vi "Get Routine Object.vi"(7 "Settings":T2=enum."Custom", 8 "error in (no error)":errorcluster, 11 "Routine":T1=enum."Secure Syringe") -> (0 "error out":errorcluster, 3 "Routine out":refnum<class "Routine.lvclass">)   [LabVIEW 2020, in "Routine.lvclass"]
uses:
  Routine.lvclass
  Pick and Place/Pick and Place.lvclass
  Pick and Place/Pick and Place Type.ctl
  Secure Syringe/SecureRelease Syringe.lvclass
  Settings.ctl
  Projects/Sensor Dispense.lvclass
  Dispense/Iterative Dispense/Iterative Dispense.lvclass
  Routine Enum.ctl
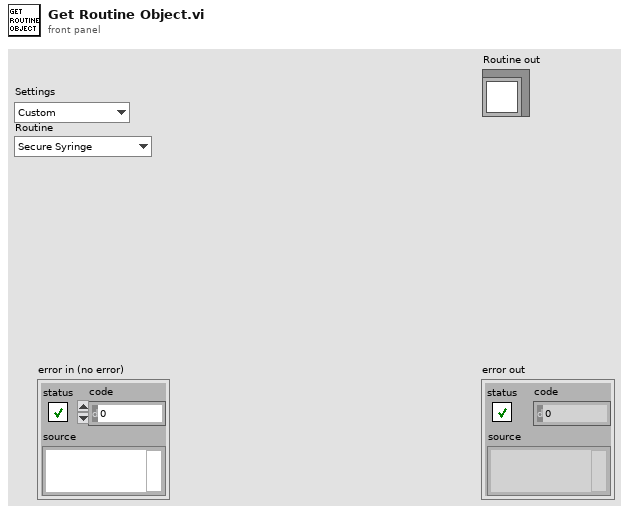
[diagram p1: front panel]
types:
  T1 = typedef "Routine.lvclass/Routine Enum.ctl" = enum16{"Primary Pick Up", "Pick Up All", "Put Down Secondary", "Put Down All", "Release Syringe", "Secondary Pick Up", "Secure Syringe", "Dispense on Plate", "Dispense on Kapton", "Dispense on Sensor"}
  T2 = typedef "Routine.lvclass/Settings.ctl" = enum16{"Default", "Custom"}
  T3 = typedef "Pick and Place.lvclass/Pick and Place Type.ctl" = enum16{"Primary Pick Up", "Secondary Pick Up", "Put Down All", "Pick Up All", "Put Down Secondary"}
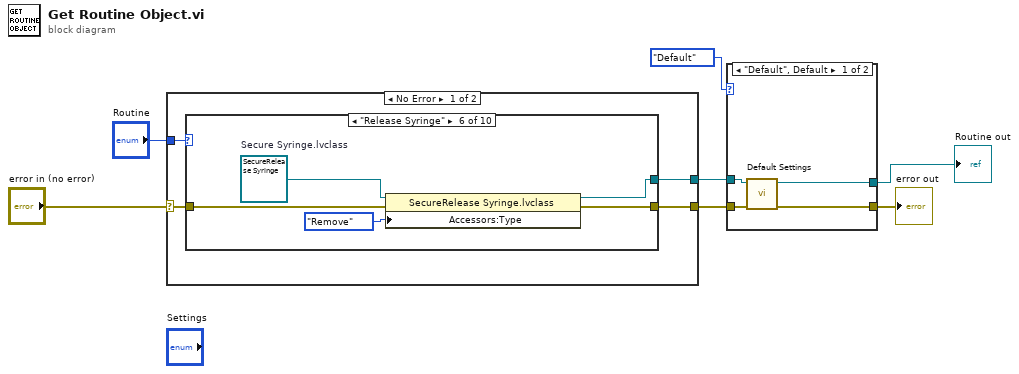
[diagram p0: block diagram]
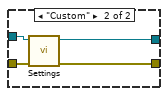
[diagram p2: hidden frame]
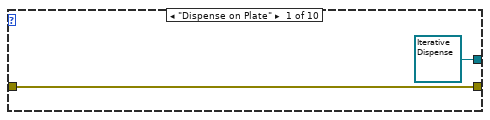
[diagram p3: hidden frame]
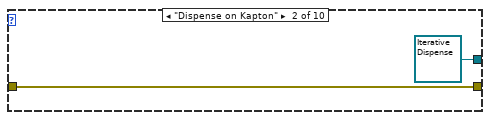
[diagram p4: hidden frame]
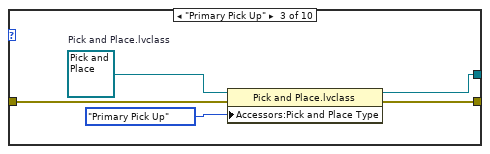
[diagram p5: hidden frame]
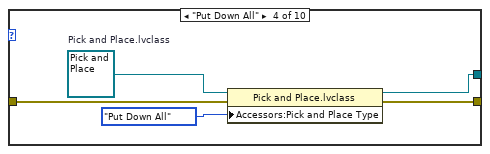
[diagram p6: hidden frame]
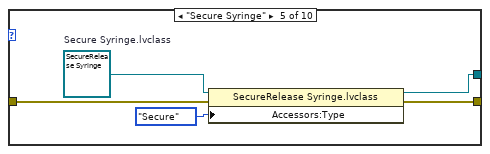
[diagram p7: hidden frame]
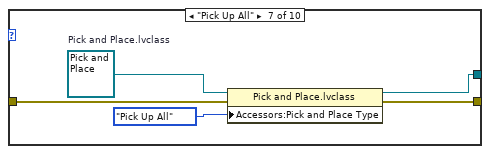
[diagram p8: hidden frame]
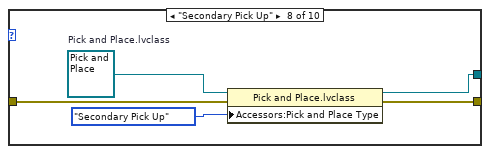
[diagram p9: hidden frame]
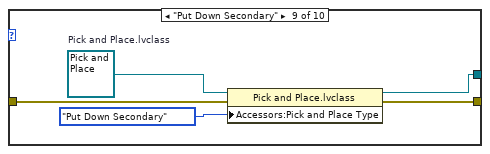
[diagram p10: hidden frame]
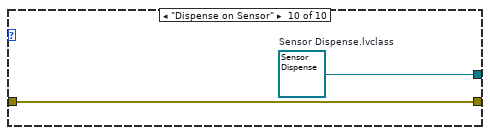
[diagram p11: hidden frame]
diagram:
  n1 = case shown="No Error" "error in (no error)" {
    selector: "error in (no error)" -> [w9 w53]
    tunnel: [w8 w53] -> w2
    tunnel: [w11 _] -> w6
    tunnel: "Routine" -> [w10 _]
    frame No Error {
      n2 = case shown="\"Release Syringe\"" w10 {
        tunnel: [refnum<class "Iterative Dispense.lvclass"> refnum ("Iterative Dispense.lvclass") refnum<class "Iterative Dispense.lvclass"> refnum ("Iterative Dispense.lvclass") w19 w24 w28 w33 w38 w43 w48 w52] -> w11
        tunnel: w9 -> [w13 w15 w17 w22 w27 w32 w37 w42 w47 w51]
        tunnel: [w13 w15 w16 w21 w26 w31 w36 w41 w46 w51] -> w8
        frame "Dispense on Plate" {
        }
        frame "Dispense on Kapton" {
        }
        frame "Primary Pick Up" {
          w20 = refnum<class "Pick and Place.lvclass"> refnum  # Pick and Place.lvclass
          n3 = property class="Pick and Place.lvclass"(reference=w20, error in=w17, "Accessors:Pick and Place Type"=Pick_and_Place_Type."Primary Pick Up" ("Pick and Place Type")) -> (reference out=w19:refnum<class "Pick and Place.lvclass">, error out=w16:errorcluster)
        }
        frame "Put Down All" {
          w25 = refnum<class "Pick and Place.lvclass"> refnum  # Pick and Place.lvclass
          n4 = property class="Pick and Place.lvclass"(reference=w25, error in=w22, "Accessors:Pick and Place Type"=Pick_and_Place_Type."Put Down All" ("Pick and Place Type")) -> (reference out=w24:refnum<class "Pick and Place.lvclass">, error out=w21:errorcluster)
        }
        frame "Secure Syringe" {
          w30 = refnum<class "SecureRelease Syringe.lvclass"> refnum  # Secure Syringe.lvclass
          n5 = property class="SecureRelease Syringe.lvclass"(reference=w30, error in=w27, "Accessors:Type"=enum16{"Secure", "Remove"}."Secure" ("Type")) -> (reference out=w28:refnum<class "SecureRelease Syringe.lvclass">, error out=w26:errorcluster)
        }
        frame "Release Syringe" {
          w35 = refnum<class "SecureRelease Syringe.lvclass"> refnum  # Secure Syringe.lvclass
          n6 = property class="SecureRelease Syringe.lvclass"(reference=w35, error in=w32, "Accessors:Type"=enum16{"Secure", "Remove"}."Remove" ("Type")) -> (reference out=w33:refnum<class "SecureRelease Syringe.lvclass">, error out=w31:errorcluster)
        }
        frame "Pick Up All" {
          w40 = refnum<class "Pick and Place.lvclass"> refnum  # Pick and Place.lvclass
          n7 = property class="Pick and Place.lvclass"(reference=w40, error in=w37, "Accessors:Pick and Place Type"=Pick_and_Place_Type."Pick Up All" ("Pick and Place Type")) -> (reference out=w38:refnum<class "Pick and Place.lvclass">, error out=w36:errorcluster)
        }
        frame "Secondary Pick Up" {
          w45 = refnum<class "Pick and Place.lvclass"> refnum  # Pick and Place.lvclass
          n8 = property class="Pick and Place.lvclass"(reference=w45, error in=w42, "Accessors:Pick and Place Type"=Pick_and_Place_Type."Secondary Pick Up" ("Pick and Place Type")) -> (reference out=w43:refnum<class "Pick and Place.lvclass">, error out=w41:errorcluster)
        }
        frame "Put Down Secondary" {
          w50 = refnum<class "Pick and Place.lvclass"> refnum  # Pick and Place.lvclass
          n9 = property class="Pick and Place.lvclass"(reference=w50, error in=w47, "Accessors:Pick and Place Type"=Pick_and_Place_Type."Put Down Secondary" ("Pick and Place Type")) -> (reference out=w48:refnum<class "Pick and Place.lvclass">, error out=w46:errorcluster)
        }
        frame "Dispense on Sensor" {
          w52 = refnum<class "Sensor Dispense.lvclass"> refnum  # Sensor Dispense.lvclass
        }
      }
    }
    frame Error {
    }
  }
  n10 = case shown="\"Default\", Default" Settings."Default" ("Settings") {
    tunnel: w6 -> [w56 w60]
    tunnel: [w57 w61] -> w5
    tunnel: w2 -> [w55 w59]
    tunnel: [w54 w58] -> w1
    frame "Default", Default {
      n11 = call-dynamic "Default Settings.vi"("error in (no error)"=w55, "Routine in"=w56) -> ("error out"=w54:errorcluster, "Routine out"=w57:refnum<class "Routine.lvclass">)  [unwired: 8 in]
    }
    frame "Custom" {
      n12 = call-dynamic "Settings.vi"("error in (no error)"=w59, "Routine in"=w60) -> ("error out"=w58:errorcluster, "Routine out"=w61:refnum<class "Routine.lvclass">)  [unwired: 8 in]
    }
  }
  "error out" <- w1
  "Routine out" <- w5
